vi "Velocity Converter- dx-dy to magnitude-heading.vi"(11 "Vector In":T2) -> (2 "Magnitude Out":dbl, 3 "Heading Out":T1 format="%05.1f")   [LabVIEW 2011]
doc: "Converts velocity in the Direction/Speed format (as defined in the appropriate Typedef) to X/Y velocity, which is the standard type within our architecture."
uses:
  2 Typedefs/Velocity.ctl
  2 Typedefs/heading.ctl
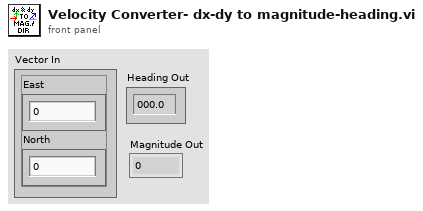
[diagram p1: front panel]
types:
  T1 = typedef "heading.ctl" = dbl
  T2 = typedef "Velocity.ctl" = cluster{"East":dbl, "North":dbl}
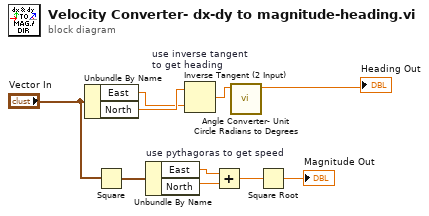
[diagram p0: block diagram]
diagram:
  n1 = Unbundle By Name("Vector In") -> ("East"=w8:dbl, "North"=w10:dbl)
  n2 = Square(x="Vector In") -> (x^2=w6:T2)
  n3 = Unbundle By Name "use pythagoras to get speed"(w6) -> ("East"=w5:dbl, "North"=w4:dbl)
  n4 = Inverse Tangent (2 Input) "use inverse tangent\nto get heading"(1:w8, 2:w10) -> (0:w9:dbl)
  n5 = Add(x=w5, y=w4) -> (x+y=w3:dbl)
  n6 = call "Angle Converter- Unit Circle Radians to Degrees.vi"("Angle in \nUnit Circle\nRadians"=w9) -> ("Angle in \nHeading \nFormat"=→"Heading Out":T1)  [unwired: 10 in]
  n7 = Square Root(x=w3) -> (sqrt(x)=→"Magnitude Out":dbl)
